vi "State_Machine.vi"(8 "error in (no error)":errorcluster caption="entrée d'erreur (pas d'erreur)", 11 "Flash_AVRDUDE en entrée":refnum<class "Flash_AVRDUDE.lvclass">) -> (0 "error out":errorcluster caption="sortie d'erreur", 2 "Json_String":string, 3 "Flash_AVRDUDE en sortie":refnum<class "Flash_AVRDUDE.lvclass">)   [LabVIEW 2020, in "Library Test.lvlib" / "Flash_AVRDUDE.lvclass"]
uses:
  Flash_AVRDUDE.lvclass
  C:/Users/ngarcin/OneDrive - Altyor/Standard TB/Class/Test/Test (Default)/Test (Default).lvclass
  Flash_AVRDUDE.lvclass/Flash_AVRDUDE.ctl
panel:
  out "String In progress":string
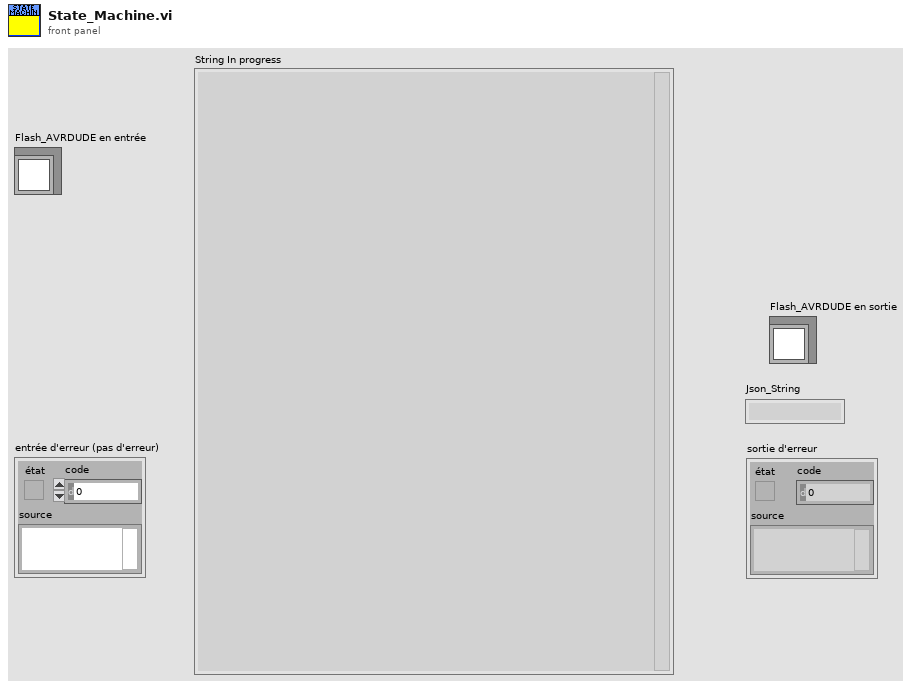
[diagram p1: front panel]
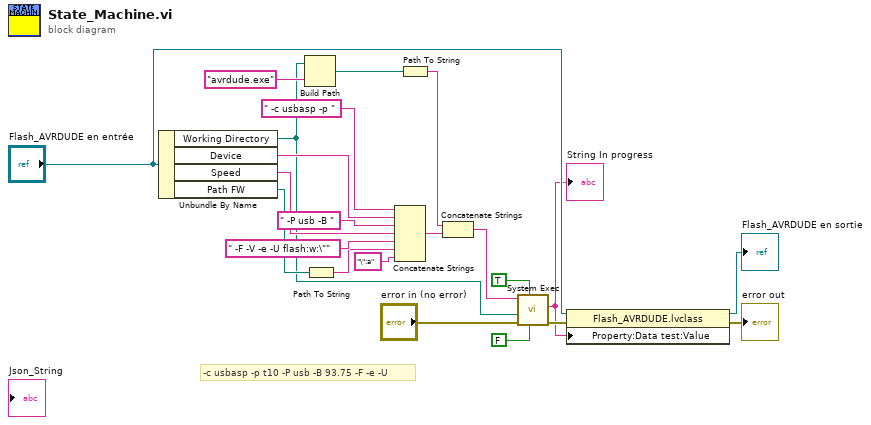
[diagram p0: block diagram]
diagram:
  # "-c usbasp -p t10 -P usb -B 93.75 -F -e -U"
  n1 = Unbundle By Name("Flash_AVRDUDE en entrée") -> ("Working Directory"=w7:path, "Device"=w9:string, "Speed"=w8:string, "Path FW"=w10:path)
  n2 = Build Path(base path=w7, name or relative path="avrdude.exe" ("nom ou chemin relatif")) -> (appended path=w22:path)
  n3 = Path To String(path=w10) -> (string=w18:string)
  n4 = Concatenate Strings(" -c usbasp -p " ("FileName"), w9, " -P usb -B " ("FileName"), w8, " -F -V -e -U flash:w:\"" ("FileName"), w18, "\":a" ("chaîne")) -> (w13:string)
  n5 = Path To String(path=w22) -> (string=w12:string)
  n6 = Concatenate Strings(w12, w13) -> (w11:string)
  n7 = call <vilib>:"System Exec.vi"("run minimized? (F)"=FALSE, "wait until completion? (T)"=TRUE, "error in (no error)"="error in (no error)", "working directory"=w7, "command line"=w11) -> ("error out"=w2:errorcluster, "standard error"=w1:string)  [unwired: 3 in, 2 out]
  "String In progress" <- w1
  n8 = property class="Flash_AVRDUDE.lvclass"(reference="Flash_AVRDUDE en entrée", error in=w2, "Property:Data test:Value"=w1) -> (reference out=→"Flash_AVRDUDE en sortie":refnum<class "Flash_AVRDUDE.lvclass">, error out=→"error out":errorcluster)
